vi "CSPP_MM.vi"(8 "error in (no error)":errorcluster) -> (0 "error out":errorcluster)   [LabVIEW 2014]
doc: "GUI for the original Actor Framework Message Maker."
uses:
  _CSPP_MessageMaker/CSPP_MessageMakerMain/CS++MessageMakerMain.lvclass
  _CSPP_MessageMaker/CSPP_MessageMakerMain/CS++MessageMakerMain.lvclass/CS++MessageMakerMain.ctl
  _CSPP_MessageMaker/CSPP_MessageMakerMain/BuildType.ctl
  <vilib>/Utility/error.llb/Error Cluster From Error Code.vi
  <vilib>/ErrorRing/Error Ring.xnode
panel:
  in  "Build Selected (Dialog&PV)":bool
  in  "Build Selected (Dialog)":bool
  in  "Build Selected (PV)":bool
  out "Progress Bar":u8(slide) scale=0.0..100.0
  out "None Found":string="No Actor classes found in this project."
  in  "Close":bool
  in  "Help":bool
  in  "Actor classes and their methods:":string[](tree)=["CS++PVProxy.lvlib:CS++PVProxy.lvclass", "CS++SVMonitor.lvlib:CS++SVMonitor.lvclass", "CS++PVMonitor.lvlib:CS++PVMonitor.lvclass", "CS++DeviceActor.lvlib:CS++DeviceActor.lvclass"]
  in  "Build Selected (simple)":bool
  in  "Projects":u16(ring) caption="Project to display:"
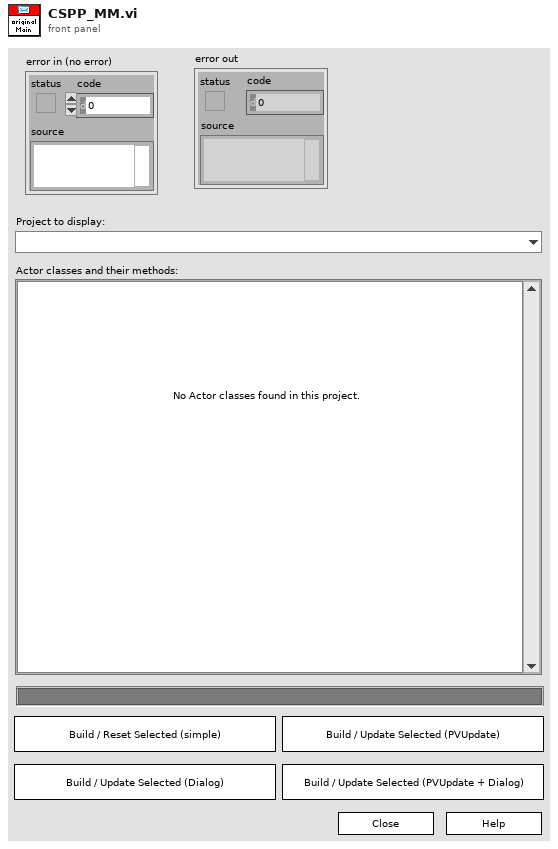
[diagram p1: front panel]
types:
  T1 = cluster{"NumberOfMessages":u16, "ActMessage":u16, "ProgressBar Notifier":refnum<notifier>}
  T2 = typedef "CS++MessageMakerMain.lvlib/CS++MessageMakerMain.lvclass/BuildType.ctl" = u16
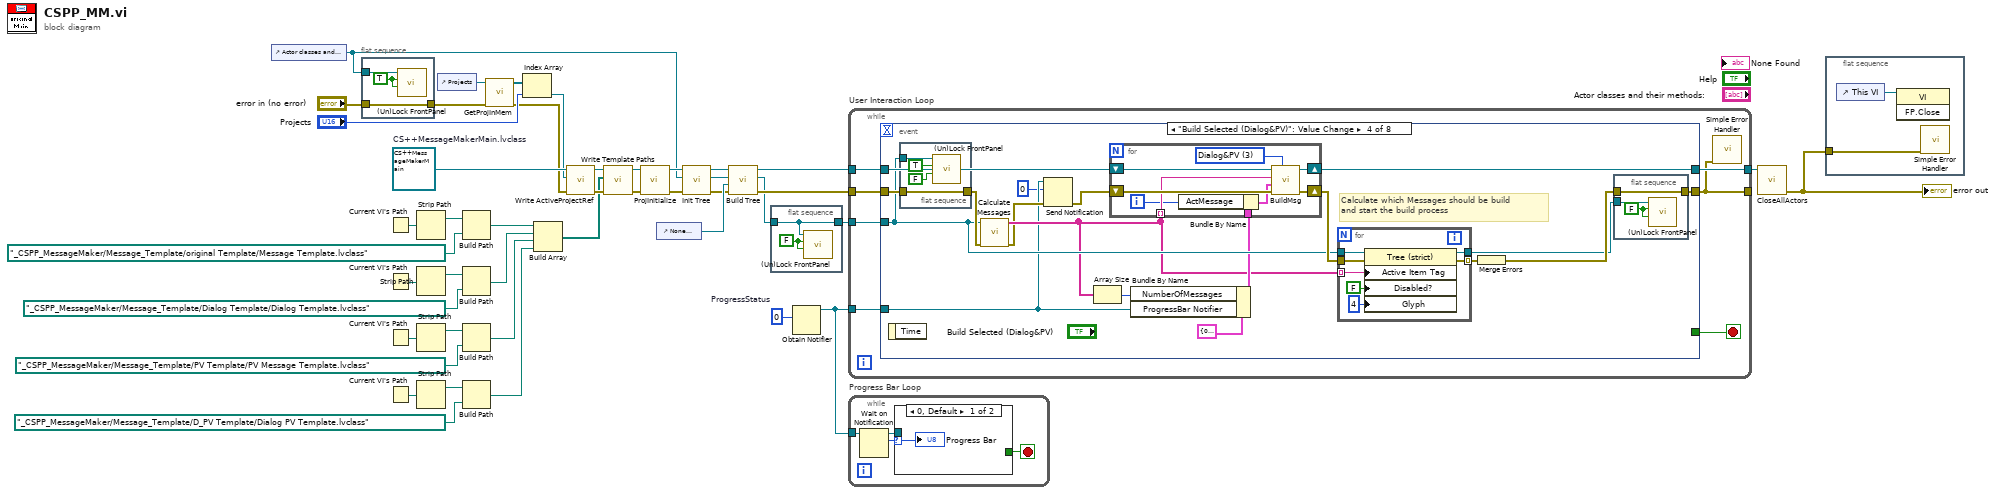
[diagram p0: block diagram]
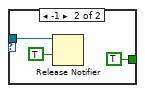
[diagram p2: hidden frame]
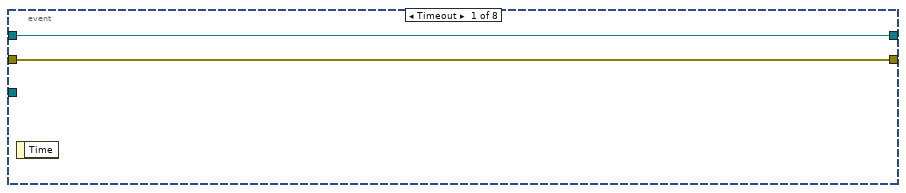
[diagram p3: hidden frame]
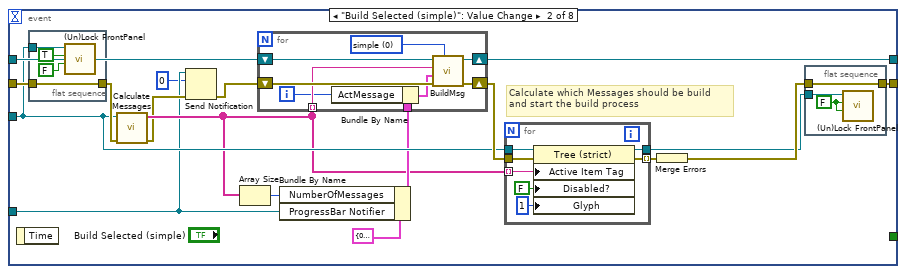
[diagram p4: hidden frame]
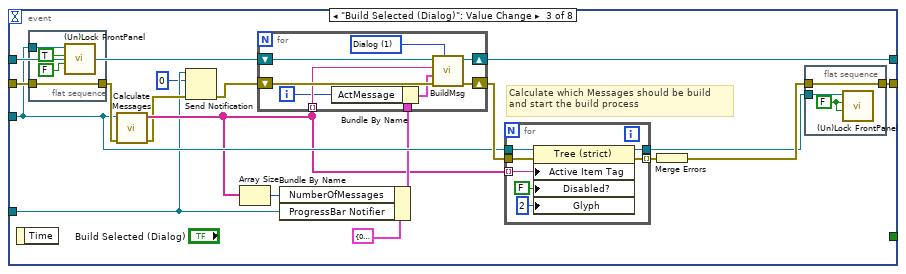
[diagram p5: hidden frame]
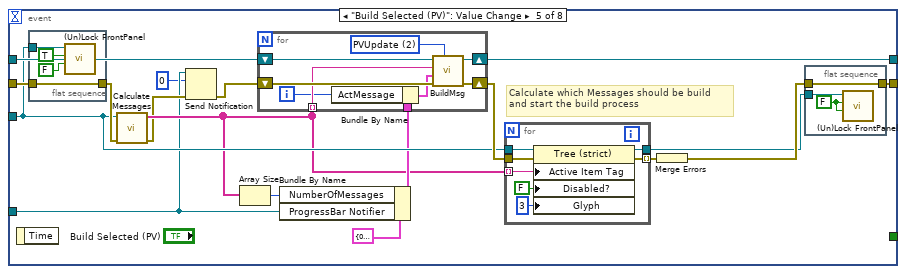
[diagram p6: hidden frame]
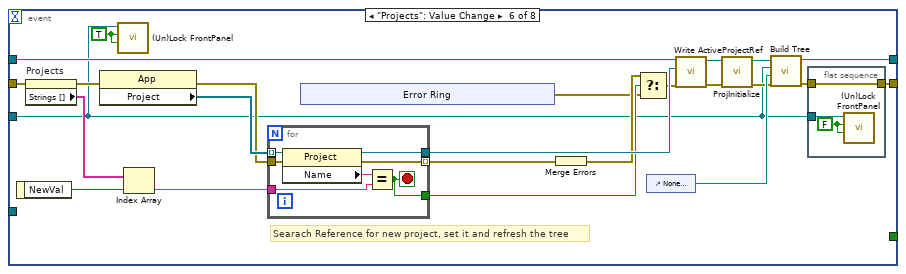
[diagram p7: hidden frame]
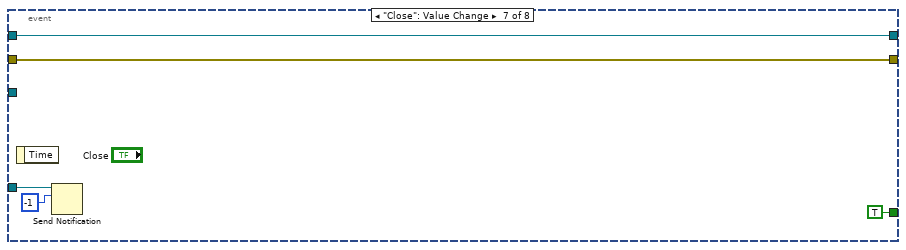
[diagram p8: hidden frame]
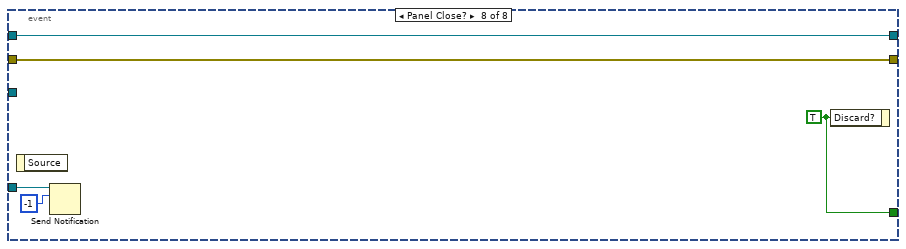
[diagram p9: hidden frame]
diagram:
  w23 = i16 0  # ProgressStatus
  w44 = refnum<class "CS++MessageMakerMain.lvclass"> refnum  # CS++MessageMakerMain.lvclass
  n1 = control-ref of="Actor classes and their methods:"() -> (w26:refnum<vi>)
  n2 = flat-sequence {
    tunnel: w26 -> [w47]
    tunnel: "error in (no error)" -> [w46]
    tunnel: [w46] -> w24
    frame #0 {
      w45 = TRUE
      n3 = call "(Un)Lock FrontPanel.vi"("SetDeferPanel?"=w45, "Lock?"=w45, "Tree Reference"=w47) -> ()  [unwired: 9 in]
    }
  }
  n4 = Current VI's Path() -> (path=w21:path)
  n5 = Current VI's Path() -> (path=w12:path)
  n6 = Current VI's Path() -> (path=w9:path)
  n7 = Current VI's Path() -> (path=w7:path)
  n8 = Strip Path(path=w21) -> (stripped path=w19:path)  [unwired: 1 out]
  n9 = Strip Path(path=w12) -> (stripped path=w11:path)  [unwired: 1 out]
  n10 = Strip Path(path=w9) -> (stripped path=w8:path)  [unwired: 1 out]
  n11 = Strip Path(path=w7) -> (stripped path=w6:path)  [unwired: 1 out]
  n12 = control-ref of="Projects"() -> (w43:refnum<vi>)
  n13 = Build Path(base path=w19, name or relative path=path "_CSPP_MessageMaker/Message_Template/original Template/Message Template.lvclass" ("Template Path")) -> (appended path=w14:path)
  n14 = Build Path(base path=w11, name or relative path=path "_CSPP_MessageMaker/Message_Template/Dialog Template/Dialog Template.lvclass" ("Template Path")) -> (appended path=w10:path)
  n15 = Build Path(base path=w8, name or relative path=path "_CSPP_MessageMaker/Message_Template/PV Template/PV Message Template.lvclass" ("Template Path")) -> (appended path=w4:path)
  n16 = Build Path(base path=w6, name or relative path=path "_CSPP_MessageMaker/Message_Template/D_PV Template/Dialog PV Template.lvclass" ("Template Path")) -> (appended path=w3:path)
  n17 = call "GetProjInMem.vi"("error in (no error)"=w24, "Ring refnum"=w43) -> ("error out"=w39:errorcluster, "Project:Projects[]"=w42:refnum<vi>[])  [unwired: 8 in]
  n18 = Index Array(array=w42, index="Projects") -> (element=w40:refnum<vi>)
  n19 = Build Array(w14, w10, w4, w3) -> (w13:path[])
  n20 = call "Write ActiveProjectRef.vi"("error in (no error)"=w39, "ActiveProjectRef"=w40, "CS++MessageMakerMain in"=w44) -> ("error out"=w18:errorcluster, "CS++MessageMakerMain out"=w16:refnum<class "CS++MessageMakerMain.lvclass">)  [unwired: 7 in]
  n21 = call "Write Template Paths.vi"("error in (no error)"=w18, "Template Paths"=w13, "CS++MessageMakerMain in"=w16) -> ("error out"=w17:errorcluster, "CS++MessageMakerMain out"=w15:refnum<class "CS++MessageMakerMain.lvclass">)  [unwired: 7 in]
  n22 = call-dynamic "ProjInitialize.vi"("error in (no error)"=w17, "CS++MessageMakerMain in"=w15) -> ("error out"=w28:errorcluster, "CS++MessageMakerMain out"=w30:refnum<class "CS++MessageMakerMain.lvclass">)  [unwired: 8 in]
  n23 = control-ref of="None Found"() -> (w35:refnum<vi>)
  n24 = call "Init Tree.vi"("error in (no error)"=w28, "Tree Reference In"=w26, "CS++MessageMakerMain in"=w30) -> ("error out"=w31:errorcluster, "Tree Reference Out"=w27:refnum<vi>, "CS++MessageMakerMain out"=w29:refnum<class "CS++MessageMakerMain.lvclass">)  [unwired: 6 in]
  n25 = call "Build Tree.vi"("error in (no error)"=w31, "No Project Text Reference"=w35, "Tree Reference In"=w27, "CS++MessageMakerMain in"=w29) -> ("error out"=w34:errorcluster, "Tree Reference Out"=w32:refnum<vi>, "CS++MessageMakerMain out"=w36:refnum<class "CS++MessageMakerMain.lvclass">)  [unwired: 5 in]
  n26 = flat-sequence {
    tunnel: [w48] -> w33
    tunnel: w32 -> [w48]
    frame #0 {
      w49 = FALSE
      n27 = call "(Un)Lock FrontPanel.vi"("SetDeferPanel?"=w49, "Lock?"=w49, "Tree Reference"=w48) -> ()  [unwired: 9 in]
    }
  }
  n28 = Obtain Notifier(notification data type=w23) -> (notifier out=w22:refnum<notifier>)  [unwired: 3 in, 2 out]
  n29 = while "User Interaction Loop" {
    tunnel: w36 -> [w52]
    tunnel: [w54] -> w37
    tunnel: w33 -> [w53]
    tunnel: w22 -> [w51]
    tunnel: w34 -> [w56]
    tunnel: [w50] -> _
    stop <- w55 stop-if-true
    n30 = event shown="[3] \"Build Selected (Dialog&PV)\": Value Change" {
      selector: _ -> [_ _ _ _ _ _ _ _]
      dyn-events: _ -> [_ _ _ _ _ _ _ _]
      timeout: _ -> [_ _ _ _ _ _ _ _]
      tunnel: w56 -> [w58 w71 w112 w153 w194 w243 w265 w268]
      tunnel: [w58 w76 w117 w158 w199 w226 w265 w268] -> w50
      tunnel: [_ _ _ _ _ _ TRUE w270] -> w55
      tunnel: w52 -> [w57 w72 w113 w154 w195 w238 w263 w269]
      tunnel: [w57 w74 w115 w156 w197 w246 w263 w269] -> w54
      tunnel: w53 -> [_ w69 w110 w151 w192 w223 _ _]
      tunnel: w51 -> [_ w62 w103 w144 w185 _ w262 w267]
      event Timeout {
        n31 = event-data() -> ()  [unwired: 1 in, 1 out]
      }
      event "Build Selected (simple)": Value Change {
        # "Calculate which Messages should be build\nand start the build process"
        n32 = event-data() -> ()  [unwired: 1 in, 1 out]
        n33 = flat-sequence {
          tunnel: w71 -> [w78]
          tunnel: [w78] -> w70
          tunnel: w69 -> [w77]
          frame #0 {
            n34 = call "(Un)Lock FrontPanel.vi"("SetDeferPanel?"=FALSE, "Lock?"=TRUE, "Tree Reference"=w77) -> ()  [unwired: 9 in]
          }
        }
        n35 = call "Calculate Messages.vi"("error in (no error)"=w70, "Tree Reference"=w69) -> ("error out"=w64:errorcluster, "Array of Messages to be build"=w67:string[])  [unwired: 8 in]
        n36 = Send Notification(notification=i16 0, notifier=w62, error in (no error)=w64) -> (error out=w63:errorcluster)  [unwired: 1 out]
        n37 = Array Size(array=w67) -> (size(s)=w66:i32)
        n38 = Bundle By Name(cluster=T1 {"NumberOfMessages"=0, "ActMessage"=0, "ProgressBar Notifier"=refnum} ("ProgressBarCluster"), "NumberOfMessages"=w66, "ProgressBar Notifier"=w62) -> (w68:T1)
        n39 = for {
          shift-right: [w93] -> w75
          shift-left: w63 -> [w95]
          shift-right: [w96] -> w74
          shift-left: w72 -> [w94]
          tunnel: w67 -> [w92] mode=indexing
          tunnel: w68 -> [w91]
          i -> [w90]
          w88 = T2 0 items=["simple", "Dialog", "PVUpdate", "Dialog&PV"] ("BuildType")
          n40 = Bundle By Name(cluster=w91, "ActMessage"=w90) -> (w89:T1)
          n41 = call "BuildMsg.vi"("BuildType"=w88, "error in (no error)"=w95, "ProgressBarCluster"=w89, "Msg to be build"=w92, "CS++MessageMakerMain in"=w94) -> ("error out"=w93:errorcluster, "CS++MessageMakerMain out"=w96:refnum<class "CS++MessageMakerMain.lvclass">)  [unwired: 5 in]
        }
        n42 = for {
          tunnel: w69 -> [w87]
          tunnel: w75 -> [w86]
          tunnel: w67 -> [w85] mode=indexing
          tunnel: [w83] -> w73 mode=indexing
          tunnel: [w82] -> w59
          n43 = property class="Tree (strict)"(reference=w87, error in=w86, "Active Item Tag"=w85, "Disabled?"=FALSE ("Active Item:Disabled?"), "Glyph"=1 ("Active Item:Symbol Index")) -> (reference out=w82:refnum<vi>, error out=w83:errorcluster)
        }
        n44 = Merge Errors(w73) -> (w60:errorcluster)
        n45 = flat-sequence {
          tunnel: [w99] -> w76
          tunnel: w60 -> [w99]
          tunnel: w59 -> [w97]
          frame #0 {
            w98 = FALSE
            n46 = call "(Un)Lock FrontPanel.vi"("SetDeferPanel?"=w98, "Lock?"=w98, "Tree Reference"=w97) -> ()  [unwired: 9 in]
          }
        }
      }
      event "Build Selected (Dialog)": Value Change {
        # "Calculate which Messages should be build\nand start the build process"
        n47 = event-data() -> ()  [unwired: 1 in, 1 out]
        n48 = flat-sequence {
          tunnel: w112 -> [w119]
          tunnel: [w119] -> w111
          tunnel: w110 -> [w118]
          frame #0 {
            n49 = call "(Un)Lock FrontPanel.vi"("SetDeferPanel?"=FALSE, "Lock?"=TRUE, "Tree Reference"=w118) -> ()  [unwired: 9 in]
          }
        }
        n50 = call "Calculate Messages.vi"("error in (no error)"=w111, "Tree Reference"=w110) -> ("error out"=w105:errorcluster, "Array of Messages to be build"=w108:string[])  [unwired: 8 in]
        n51 = Send Notification(notification=i16 0, notifier=w103, error in (no error)=w105) -> (error out=w104:errorcluster)  [unwired: 1 out]
        n52 = Array Size(array=w108) -> (size(s)=w107:i32)
        n53 = Bundle By Name(cluster=T1 {"NumberOfMessages"=0, "ActMessage"=0, "ProgressBar Notifier"=refnum} ("ProgressBarCluster"), "NumberOfMessages"=w107, "ProgressBar Notifier"=w103) -> (w109:T1)
        n54 = for {
          shift-right: [w134] -> w116
          shift-left: w104 -> [w136]
          shift-right: [w137] -> w115
          shift-left: w113 -> [w135]
          tunnel: w108 -> [w133] mode=indexing
          tunnel: w109 -> [w132]
          i -> [w131]
          w129 = T2 1 items=["simple", "Dialog", "PVUpdate", "Dialog&PV"] ("BuildType")
          n55 = Bundle By Name(cluster=w132, "ActMessage"=w131) -> (w130:T1)
          n56 = call "BuildMsg.vi"("BuildType"=w129, "error in (no error)"=w136, "ProgressBarCluster"=w130, "Msg to be build"=w133, "CS++MessageMakerMain in"=w135) -> ("error out"=w134:errorcluster, "CS++MessageMakerMain out"=w137:refnum<class "CS++MessageMakerMain.lvclass">)  [unwired: 5 in]
        }
        n57 = for {
          tunnel: w110 -> [w128]
          tunnel: w116 -> [w127]
          tunnel: w108 -> [w126] mode=indexing
          tunnel: [w124] -> w114 mode=indexing
          tunnel: [w123] -> w100
          n58 = property class="Tree (strict)"(reference=w128, error in=w127, "Active Item Tag"=w126, "Disabled?"=FALSE ("Active Item:Disabled?"), "Glyph"=2 ("Active Item:Symbol Index")) -> (reference out=w123:refnum<vi>, error out=w124:errorcluster)
        }
        n59 = Merge Errors(w114) -> (w101:errorcluster)
        n60 = flat-sequence {
          tunnel: [w140] -> w117
          tunnel: w101 -> [w140]
          tunnel: w100 -> [w138]
          frame #0 {
            w139 = FALSE
            n61 = call "(Un)Lock FrontPanel.vi"("SetDeferPanel?"=w139, "Lock?"=w139, "Tree Reference"=w138) -> ()  [unwired: 9 in]
          }
        }
      }
      event "Build Selected (Dialog&PV)": Value Change {
        # "Calculate which Messages should be build\nand start the build process"
        n62 = event-data() -> ()  [unwired: 1 in, 1 out]
        n63 = flat-sequence {
          tunnel: w153 -> [w160]
          tunnel: [w160] -> w152
          tunnel: w151 -> [w159]
          frame #0 {
            n64 = call "(Un)Lock FrontPanel.vi"("SetDeferPanel?"=FALSE, "Lock?"=TRUE, "Tree Reference"=w159) -> ()  [unwired: 9 in]
          }
        }
        n65 = call "Calculate Messages.vi"("error in (no error)"=w152, "Tree Reference"=w151) -> ("error out"=w146:errorcluster, "Array of Messages to be build"=w149:string[])  [unwired: 8 in]
        n66 = Send Notification(notification=i16 0, notifier=w144, error in (no error)=w146) -> (error out=w145:errorcluster)  [unwired: 1 out]
        n67 = Array Size(array=w149) -> (size(s)=w148:i32)
        n68 = Bundle By Name(cluster=T1 {"NumberOfMessages"=0, "ActMessage"=0, "ProgressBar Notifier"=refnum} ("ProgressBarCluster"), "NumberOfMessages"=w148, "ProgressBar Notifier"=w144) -> (w150:T1)
        n69 = for {
          shift-right: [w175] -> w157
          shift-left: w145 -> [w177]
          shift-right: [w178] -> w156
          shift-left: w154 -> [w176]
          tunnel: w149 -> [w174] mode=indexing
          tunnel: w150 -> [w173]
          i -> [w172]
          w170 = T2 3 items=["simple", "Dialog", "PVUpdate", "Dialog&PV"] ("BuildType")
          n70 = Bundle By Name(cluster=w173, "ActMessage"=w172) -> (w171:T1)
          n71 = call "BuildMsg.vi"("BuildType"=w170, "error in (no error)"=w177, "ProgressBarCluster"=w171, "Msg to be build"=w174, "CS++MessageMakerMain in"=w176) -> ("error out"=w175:errorcluster, "CS++MessageMakerMain out"=w178:refnum<class "CS++MessageMakerMain.lvclass">)  [unwired: 5 in]
        }
        n72 = for {
          tunnel: w151 -> [w169]
          tunnel: w157 -> [w168]
          tunnel: w149 -> [w167] mode=indexing
          tunnel: [w165] -> w155 mode=indexing
          tunnel: [w164] -> w141
          n73 = property class="Tree (strict)"(reference=w169, error in=w168, "Active Item Tag"=w167, "Disabled?"=FALSE ("Active Item:Disabled?"), "Glyph"=4 ("Active Item:Symbol Index")) -> (reference out=w164:refnum<vi>, error out=w165:errorcluster)
        }
        n74 = Merge Errors(w155) -> (w142:errorcluster)
        n75 = flat-sequence {
          tunnel: [w181] -> w158
          tunnel: w142 -> [w181]
          tunnel: w141 -> [w179]
          frame #0 {
            w180 = FALSE
            n76 = call "(Un)Lock FrontPanel.vi"("SetDeferPanel?"=w180, "Lock?"=w180, "Tree Reference"=w179) -> ()  [unwired: 9 in]
          }
        }
      }
      event "Build Selected (PV)": Value Change {
        # "Calculate which Messages should be build\nand start the build process"
        n77 = event-data() -> ()  [unwired: 1 in, 1 out]
        n78 = flat-sequence {
          tunnel: w194 -> [w201]
          tunnel: [w201] -> w193
          tunnel: w192 -> [w200]
          frame #0 {
            n79 = call "(Un)Lock FrontPanel.vi"("SetDeferPanel?"=FALSE, "Lock?"=TRUE, "Tree Reference"=w200) -> ()  [unwired: 9 in]
          }
        }
        n80 = call "Calculate Messages.vi"("error in (no error)"=w193, "Tree Reference"=w192) -> ("error out"=w187:errorcluster, "Array of Messages to be build"=w190:string[])  [unwired: 8 in]
        n81 = Send Notification(notification=i16 0, notifier=w185, error in (no error)=w187) -> (error out=w186:errorcluster)  [unwired: 1 out]
        n82 = Array Size(array=w190) -> (size(s)=w189:i32)
        n83 = Bundle By Name(cluster=T1 {"NumberOfMessages"=0, "ActMessage"=0, "ProgressBar Notifier"=refnum} ("ProgressBarCluster"), "NumberOfMessages"=w189, "ProgressBar Notifier"=w185) -> (w191:T1)
        n84 = for {
          shift-right: [w216] -> w198
          shift-left: w186 -> [w218]
          shift-right: [w219] -> w197
          shift-left: w195 -> [w217]
          tunnel: w190 -> [w215] mode=indexing
          tunnel: w191 -> [w214]
          i -> [w213]
          w211 = T2 2 items=["simple", "Dialog", "PVUpdate", "Dialog&PV"] ("BuildType")
          n85 = Bundle By Name(cluster=w214, "ActMessage"=w213) -> (w212:T1)
          n86 = call "BuildMsg.vi"("BuildType"=w211, "error in (no error)"=w218, "ProgressBarCluster"=w212, "Msg to be build"=w215, "CS++MessageMakerMain in"=w217) -> ("error out"=w216:errorcluster, "CS++MessageMakerMain out"=w219:refnum<class "CS++MessageMakerMain.lvclass">)  [unwired: 5 in]
        }
        n87 = for {
          tunnel: w192 -> [w210]
          tunnel: w198 -> [w209]
          tunnel: w190 -> [w208] mode=indexing
          tunnel: [w206] -> w196 mode=indexing
          tunnel: [w205] -> w182
          n88 = property class="Tree (strict)"(reference=w210, error in=w209, "Active Item Tag"=w208, "Disabled?"=FALSE ("Active Item:Disabled?"), "Glyph"=3 ("Active Item:Symbol Index")) -> (reference out=w205:refnum<vi>, error out=w206:errorcluster)
        }
        n89 = Merge Errors(w196) -> (w183:errorcluster)
        n90 = flat-sequence {
          tunnel: [w222] -> w199
          tunnel: w183 -> [w222]
          tunnel: w182 -> [w220]
          frame #0 {
            w221 = FALSE
            n91 = call "(Un)Lock FrontPanel.vi"("SetDeferPanel?"=w221, "Lock?"=w221, "Tree Reference"=w220) -> ()  [unwired: 9 in]
          }
        }
      }
      event "Projects": Value Change {
        w224 = TRUE
        # "Searach Reference for new project, set it and refresh the tree"
        n92 = event-data() -> ("NewVal"=w241:u16)  [unwired: 1 in]
        n93 = property on="Projects" class="Ring (strict)"(error in=w243) -> (error out=w227:errorcluster, "Strings []"=w242:string[])  [unwired: 1 in, 1 out]
        n94 = property class="App"(error in=w227) -> (error out=w244:errorcluster, "Project"=w245:refnum<vi>[])  [unwired: 1 in, 1 out]
        n95 = call "(Un)Lock FrontPanel.vi"("SetDeferPanel?"=w224, "Lock?"=w224, "Tree Reference"=w223) -> ()  [unwired: 9 in]
        n96 = Index Array(array=w242, index=w241) -> (element=w240:string)
        n97 = for {
          tunnel: w245 -> [w260] mode=indexing
          tunnel: w244 -> [w259]
          tunnel: [w258] -> w236 mode=indexing
          tunnel: [w256] -> w239
          tunnel: w240 -> [w255]
          tunnel: [w254] -> w237
          stop <- w254 stop-if-true
          n98 = property class="Project"(reference=w260, error in=w259) -> (reference out=w256:refnum<vi>, error out=w258:errorcluster, "Name"=w257:string)
          n99 = Equal?(x=w257, y=w255) -> (x = y?=w254:bool)
        }
        n100 = xnode "Error Ring"() -> ("error out"=w234:errorcluster)
        n101 = Merge Errors(w236) -> (w235:errorcluster)
        n102 = Select(t=w235, s=w237, f=w234) -> (s? t:f=w233:errorcluster)
        n103 = control-ref of="None Found"() -> (w232:refnum<vi>)
        n104 = call "Write ActiveProjectRef.vi"("error in (no error)"=w233, "ActiveProjectRef"=w239, "CS++MessageMakerMain in"=w238) -> ("error out"=w229:errorcluster, "CS++MessageMakerMain out"=w231:refnum<class "CS++MessageMakerMain.lvclass">)  [unwired: 7 in]
        n105 = call-dynamic "ProjInitialize.vi"("error in (no error)"=w229, "CS++MessageMakerMain in"=w231) -> ("error out"=w228:errorcluster, "CS++MessageMakerMain out"=w230:refnum<class "CS++MessageMakerMain.lvclass">)  [unwired: 8 in]
        n106 = call "Build Tree.vi"("error in (no error)"=w228, "No Project Text Reference"=w232, "Tree Reference In"=w223, "CS++MessageMakerMain in"=w230) -> ("error out"=w225:errorcluster, "CS++MessageMakerMain out"=w246:refnum<class "CS++MessageMakerMain.lvclass">)  [unwired: 5 in, 1 out]
        n107 = flat-sequence {
          tunnel: [w249] -> w226
          tunnel: w225 -> [w249]
          tunnel: w223 -> [w247]
          frame #0 {
            w248 = FALSE
            n108 = call "(Un)Lock FrontPanel.vi"("SetDeferPanel?"=w248, "Lock?"=w248, "Tree Reference"=w247) -> ()  [unwired: 9 in]
          }
        }
      }
      event "Close": Value Change {
        n109 = event-data() -> ()  [unwired: 1 in, 1 out]
        n110 = Send Notification(notification=i16 -1, notifier=w262) -> ()  [unwired: 1 in, 2 out]
      }
      event Panel Close? {
        w270 = TRUE ("Discard?")
        n111 = event-data() -> ()  [unwired: 1 in, 1 out]
        n112 = Send Notification(notification=i16 -1, notifier=w267) -> ()  [unwired: 1 in, 2 out]
        n113 = event-data("Discard?"=w270) -> ()  [unwired: 1 in, 1 out]
      }
    }
    n114 = call <vilib>:"Simple Error Handler.vi"("error in (no error)"=w50) -> ()  [unwired: 4 in, 5 out]
  }
  n115 = while "Progress Bar Loop" {
    tunnel: w22 -> [w274]
    stop <- w271 stop-if-true
    n116 = Wait on Notification(notifier=w274) -> (notifier out=w272:refnum<notifier>, notification=w273:i16)  [unwired: 3 in, 2 out]
    n117 = case shown="0, Default" w273 {
      selector: w273 -> [w275 _]
      tunnel: w272 -> [_ w278]
      tunnel: [_ TRUE] -> w271
      frame 0, Default {
        "Progress Bar" <- w275
      }
      frame -1 {
        n118 = Release Notifier(notifier=w278, force destroy? (F)=TRUE) -> ()  [unwired: 1 in, 3 out]
      }
    }
  }
  n119 = call-dynamic "CloseAllActors.vi"("CS++MessageMakerMain in"=w37) -> ("error out"=w38:errorcluster)  [unwired: 9 in, 1 out]
  "error out" <- w38
  n120 = flat-sequence {
    tunnel: w38 -> [w280]
    frame #0 {
      n121 = control-ref of="This VI"() -> (w279:refnum<vi>)
      n122 = invoke class="VI" method="FP.Close"(reference=w279) -> ()  [unwired: 2 in, 3 out]
      n123 = call <vilib>:"Simple Error Handler.vi"("error in (no error)"=w280) -> ()  [unwired: 4 in, 5 out]
    }
  }
